vi "Configure Power.vi"(0 "VISA resource name":refnum<visa-resource-name>, 1 "Power Reference (0 dBm)":dbl, 2 "Enable Power Reference (F:Disable)":bool, 5 "Power (-130 dBm)":dbl=-130.0, 7 "Power Offset (0 dB)":dbl, 9 "Attenuator Auto Mode (T:Enable)":bool=TRUE, 11 "error in (no error)":errorcluster, 12 "Enable Attenuator Bypass (F:Disable)":bool, 13 "Attenuation Level (115 dB)":dbl=115.0) -> (4 "VISA resource name out":refnum<visa-resource-name>, 15 "error out":errorcluster)   [LabVIEW 2014, in "Agilent PSG MXG Series.lvlib"]
doc: "Configures RF output power."
uses:
  Agilent PSG MXG Series.lvlib
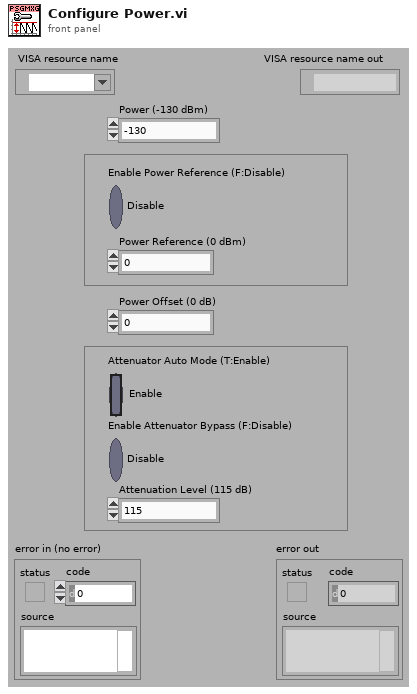
[diagram p1: front panel]
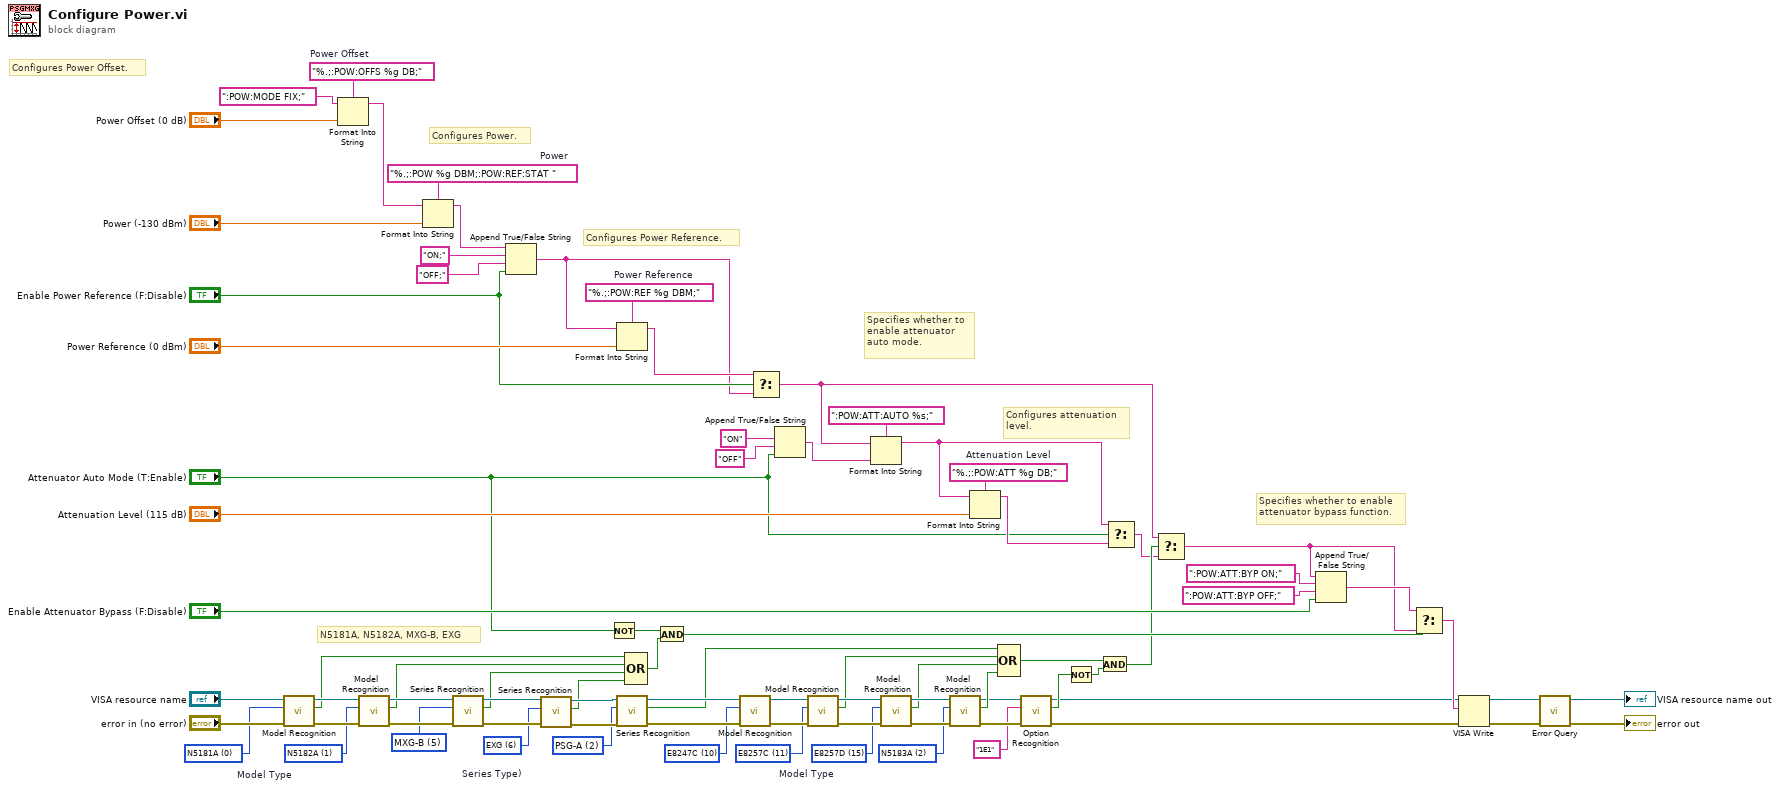
[diagram p0: block diagram]
diagram:
  w1 = u16 2 items=["N5181A"=0, "N5182A"=1, "N5183A"=2, "N5161A"=3, "N5162A"=4, "E8241A"=5, "E8244A"=6, "E8251A"=7, "E8254A"=8, "E8247C"=10, "E8257C"=11, "E8267C"=12, "E8257D"=15, "E8267D"=16, "N5171B"=17, "N5172B"=18, "N5181B"=19, "N5182B"=20] ("Model Type (0: N5181A)")
  w2 = u16 15 items=["N5181A"=0, "N5182A"=1, "N5183A"=2, "N5161A"=3, "N5162A"=4, "E8241A"=5, "E8244A"=6, "E8251A"=7, "E8254A"=8, "E8247C"=10, "E8257C"=11, "E8267C"=12, "E8257D"=15, "E8267D"=16, "N5171B"=17, "N5172B"=18, "N5181B"=19, "N5182B"=20] ("Model Type (0: N5181A)")
  w3 = u16 11 items=["N5181A"=0, "N5182A"=1, "N5183A"=2, "N5161A"=3, "N5162A"=4, "E8241A"=5, "E8244A"=6, "E8251A"=7, "E8254A"=8, "E8247C"=10, "E8257C"=11, "E8267C"=12, "E8257D"=15, "E8267D"=16, "N5171B"=17, "N5172B"=18, "N5181B"=19, "N5182B"=20] ("Model Type (0: N5181A)")
  w4 = u16 10 items=["N5181A"=0, "N5182A"=1, "N5183A"=2, "N5161A"=3, "N5162A"=4, "E8241A"=5, "E8244A"=6, "E8251A"=7, "E8254A"=8, "E8247C"=10, "E8257C"=11, "E8267C"=12, "E8257D"=15, "E8267D"=16, "N5171B"=17, "N5172B"=18, "N5181B"=19, "N5182B"=20]  # Model Type
  w5 = u16 2 items=["MXG-A", "PSG", "PSG-A", "PSG-C", "PSG-D", "MXG-B", "EXG"] ("Series Type (0: MXG)")
  w12 = u16 6 items=["MXG-A", "PSG", "PSG-A", "PSG-C", "PSG-D", "MXG-B", "EXG"] ("Series Type (0: MXG)")
  w13 = u16 5 items=["MXG-A", "PSG", "PSG-A", "PSG-C", "PSG-D", "MXG-B", "EXG"]  # Series Type)
  w20 = u16 1 items=["N5181A"=0, "N5182A"=1, "N5183A"=2, "N5161A"=3, "N5162A"=4, "E8241A"=5, "E8244A"=6, "E8251A"=7, "E8254A"=8, "E8247C"=10, "E8257C"=11, "E8267C"=12, "E8257D"=15, "E8267D"=16, "N5171B"=17, "N5172B"=18, "N5181B"=19, "N5182B"=20] ("Model Type (0: N5181A)")
  w21 = u16 0 items=["N5181A"=0, "N5182A"=1, "N5183A"=2, "N5161A"=3, "N5162A"=4, "E8241A"=5, "E8244A"=6, "E8251A"=7, "E8254A"=8, "E8247C"=10, "E8257C"=11, "E8267C"=12, "E8257D"=15, "E8267D"=16, "N5171B"=17, "N5172B"=18, "N5181B"=19, "N5182B"=20]  # Model Type
  w60 = "%.;:POW:OFFS %g DB;"  # Power Offset
  w74 = "%.;:POW:ATT %g DB;"  # Attenuation Level
  w77 = "%.;:POW:REF %g DBM;"  # Power Reference
  w82 = "%.;:POW %g DBM;:POW:REF:STAT "  # Power
  # "N5181A, N5182A, MXG-B, EXG"
  # "Specifies whether to enable\nattenuator bypass function."
  # "Configures attenuation\nlevel."
  # "Specifies whether to\nenable attenuator\nauto mode."
  # "Configures Power Offset."
  # "Configures Power Reference."
  # "Configures Power."
  n1 = call "Model Recognition.vi"("error in (no error)"="error in (no error)", "Model Type (0: N5181A)"=w21, "VISA resource name"="VISA resource name") -> ("error out"=w51:errorcluster, "Is Model Correct"=w6:bool, "VISA resource name out"=w52:refnum<visa-resource-name>)  [unwired: 6 out]
  n2 = Format Into String(format string=w60, initial string=":POW:MODE FIX;" ("Power Mode"), "Power Offset (0 dB)") -> (resulting string=w22:string)  [unwired: 1 in, 1 out]
  n3 = call "Model Recognition.vi"("error in (no error)"=w51, "Model Type (0: N5181A)"=w20, "VISA resource name"=w52) -> ("error out"=w16:errorcluster, "Is Model Correct"=w7:bool, "VISA resource name out"=w19:refnum<visa-resource-name>)  [unwired: 6 out]
  n4 = Format Into String(format string=w82, initial string=w22, "Power (-130 dBm)") -> (resulting string=w80:string)  [unwired: 1 in, 1 out]
  n5 = call "Series Recognition.vi"("error in (no error)"=w16, "Series Type (0: MXG)"=w13, "VISA resource name"=w19) -> ("error out"=w15:errorcluster, "Is Series Correct"=w8:bool, "VISA resource name out"=w18:refnum<visa-resource-name>)  [unwired: 6 out]
  n6 = Append True/False String(1:"Enable Power Reference (F:Disable)", 2:"OFF;" ("false string"), 3:"ON;" ("true string"), 4:w80) -> (0:w62:string)
  n7 = call "Series Recognition.vi"("error in (no error)"=w15, "Series Type (0: MXG)"=w12, "VISA resource name"=w18) -> ("error out"=w14:errorcluster, "Is Series Correct"=w9:bool, "VISA resource name out"=w17:refnum<visa-resource-name>)  [unwired: 6 out]
  n8 = Not(x="Attenuator Auto Mode (T:Enable)") -> (.not. x?=w11:bool)
  n9 = Format Into String(format string=w77, initial string=w62, "Power Reference (0 dBm)") -> (resulting string=w63:string)  [unwired: 1 in, 1 out]
  n10 = call "Series Recognition.vi"("error in (no error)"=w14, "Series Type (0: MXG)"=w5, "VISA resource name"=w17) -> ("error out"=w49:errorcluster, "Is Series Correct"=w42:bool, "VISA resource name out"=w50:refnum<visa-resource-name>)  [unwired: 6 out]
  n11 = Compound Arithmetic op=OR(w6, w7, w8, w9) -> (w10:bool)
  n12 = And(x=w11, y=w10) -> (x .and. y?=w65:bool)
  n13 = call "Model Recognition.vi"("error in (no error)"=w49, "Model Type (0: N5181A)"=w4, "VISA resource name"=w50) -> ("error out"=w47:errorcluster, "VISA resource name out"=w48:refnum<visa-resource-name>)  [unwired: 7 out]
  n14 = Select(t=w63, s="Enable Power Reference (F:Disable)", f=w62) -> (s? t:f=w24:string)
  n15 = Append True/False String(1:"Attenuator Auto Mode (T:Enable)", 2:"OFF" ("false string"), 3:"ON" ("true string")) -> (0:w33:string)  [unwired: 1 out]
  n16 = call "Model Recognition.vi"("error in (no error)"=w47, "Model Type (0: N5181A)"=w3, "VISA resource name"=w48) -> ("error out"=w45:errorcluster, "Is Model Correct"=w41:bool, "VISA resource name out"=w46:refnum<visa-resource-name>)  [unwired: 6 out]
  n17 = Format Into String(format string=":POW:ATT:AUTO %s;", initial string=w24, w33) -> (resulting string=w32:string)  [unwired: 1 in, 1 out]
  n18 = call "Model Recognition.vi"("error in (no error)"=w45, "Model Type (0: N5181A)"=w2, "VISA resource name"=w46) -> ("error out"=w43:errorcluster, "Is Model Correct"=w40:bool, "VISA resource name out"=w44:refnum<visa-resource-name>)  [unwired: 6 out]
  n19 = call "Model Recognition.vi"("error in (no error)"=w43, "Model Type (0: N5181A)"=w1, "VISA resource name"=w44) -> ("error out"=w37:errorcluster, "Is Model Correct"=w39:bool, "VISA resource name out"=w38:refnum<visa-resource-name>)  [unwired: 6 out]
  n20 = Format Into String(format string=w74, initial string=w32, "Attenuation Level (115 dB)") -> (resulting string=w72:string)  [unwired: 1 in, 1 out]
  n21 = Compound Arithmetic op=OR(w42, w41, w40, w39) -> (w35:bool)
  n22 = call "Option Recognition.vi"("error in (no error)"=w37, "Option (\"\")"="1E1" ("Option (\"\")"), "VISA resource name"=w38) -> ("error out"=w25:errorcluster, "Is Option Installed"=w29:bool, "VISA resource name out"=w26:refnum<visa-resource-name>)  [unwired: 6 out]
  n23 = Not(x=w29) -> (.not. x?=w30:bool)
  n24 = And(x=w35, y=w30) -> (x .and. y?=w31:bool)
  n25 = Select(t=w32, s="Attenuator Auto Mode (T:Enable)", f=w72) -> (s? t:f=w28:string)
  n26 = Select(t=w24, s=w31, f=w28) -> (s? t:f=w27:string)
  n27 = Append True/False String(1:"Enable Attenuator Bypass (F:Disable)", 2:":POW:ATT:BYP OFF;" ("true string"), 3:":POW:ATT:BYP ON;" ("true string"), 4:w27) -> (0:w57:string)
  n28 = Select(t=w57, s=w65, f=w27) -> (s? t:f=w67:string)
  n29 = VISA Write(VISA resource name=w26, write buffer=w67, error in (no error)=w25) -> (VISA resource name out=w69:refnum<visa-resource-name>, error out=w68:errorcluster)  [unwired: 1 out]
  n30 = call "Error Query.vi"("error in (no error)"=w68, "VISA resource name"=w69) -> ("error out"=→"error out":errorcluster, "VISA resource name out"=→"VISA resource name out":refnum<visa-resource-name>)  [unwired: 8 out]
